vi "parse_i32_scalar.vi"(4 "error in":errorcluster, 6 "type":i32, 7 "msg in":string) -> (0 "error out":errorcluster, 2 "number":i32, 3 "msg out":string)   [LabVIEW 2012]
doc: "Parses out a 32bit integer from msg in. The remaining string is returned in msg out."
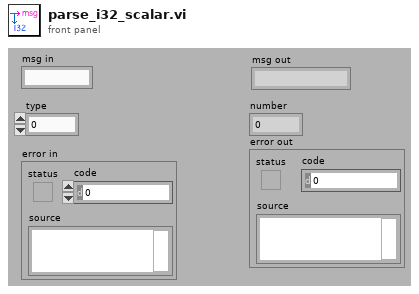
[diagram p1: front panel]
types:
  T1 = enum16{"big-endian, network order", "native, host order", "little-endian"}
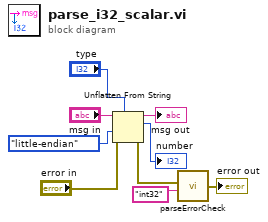
[diagram p0: block diagram]
diagram:
  n1 = Unflatten From String(type="type", binary string="msg in", byte order (0:big-endian, network order)=T1."little-endian", error in (no error)="error in") -> (rest of the binary string=→"msg out":string, value=→"number":i32, error out=w4:errorcluster)  [unwired: 1 in]
  n2 = call <userlib>:"parseErrorCheck.vi"("type"="int32", "error in"=w4) -> ("error out"=→"error out":errorcluster)  [unwired: 2 in]
